vi "DataSocket Write Connections Manager.vi"(10 "URL":string, 11 "Action":enum16{"Get", "Close", "Close All"}(ring)) -> (3 "connection id":refnum<k13>)   [LabVIEW 2023, in "Reply Msg DataSocket Connections Managed.lvclass"]
uses:
  Reply Msg DataSocket Connections Managed.lvclass
  Reply Msg DataSocket Connections Managed.lvclass/Reply Msg DataSocket Connections Managed.ctl
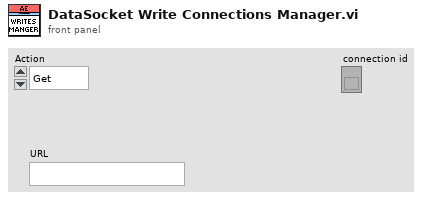
[diagram p1: front panel]
types:
  T1 = enum16{"Read", "Write", "ReadWrite", "BufferedRead", "BufferedReadWrite"}
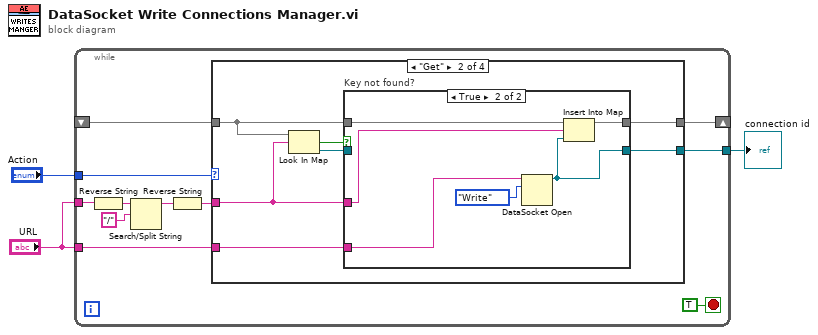
[diagram p0: block diagram]
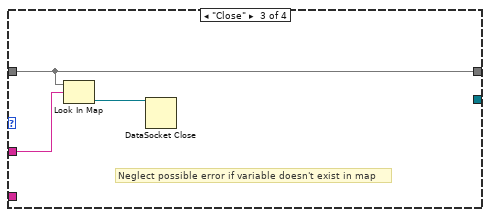
[diagram p4: hidden frame]
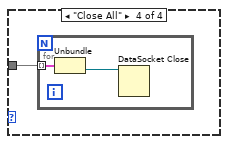
[diagram p5: hidden frame]
diagram:
  n1 = while {
    shift-right: [w12] -> _
    shift-left: _ -> [w11]
    tunnel: "URL" -> [w6]
    tunnel: [w10] -> w2
    tunnel: "Action" -> [w13]
    tunnel: "URL" -> [w4]
    stop <- TRUE stop-if-true
    n2 = Reverse String(1:w6) -> (0:w9:string)
    n3 = Search/Split String(string=w9, search string/char (-)="/") -> (substring before match=w7:string)  [unwired: 1 in, 2 out]
    n4 = Reverse String(1:w7) -> (0:w5:string)
    n5 = case shown="\"Get\"" w13 {
      tunnel: [_ w19 w30 _] -> w12
      tunnel: w11 -> [_ w20 w30 w33]
      tunnel: w5 -> [_ w18 w32 _]
      tunnel: [_ w16 _ _] -> w10
      tunnel: w4 -> [_ w15 _ _]
      frame Default {
      }
      frame "Get" {
        n6 = Look In Map(map=w20, key=w18) -> (key not found?=w21:bool, value=w17:refnum<k13>)  [unwired: 1 in]
        n7 = case "Key not found?" shown="True" w21 {
          tunnel: w20 -> [w22 w29]
          tunnel: [w22 w28] -> w19
          tunnel: w18 -> [_ w25]
          tunnel: w17 -> [w23 _]
          tunnel: [w23 w27] -> w16
          tunnel: w15 -> [_ w24]
          frame False {
          }
          frame True {
            n8 = DataSocket Open(10:T1."Write" ("mode"), 11:w24) -> (3:w27:refnum<k13>)  [unwired: 2 in, 1 out]
            n9 = Insert Into Map(map in=w29, key=w25, value=w27) -> (map out=w28:map{string, refnum<k13>})  [unwired: 2 out]
          }
        }
      }
      frame "Close" {
        # "Neglect possible error if variable doesn't exist in map"
        n10 = Look In Map(map=w30, key=w32) -> (value=w31:refnum<k13>)  [unwired: 1 in, 1 out]
        n11 = DataSocket Close(11:w31) -> ()  [unwired: 2 in, 2 out]
      }
      frame "Close All" {
        n12 = for {
          tunnel: w33 -> [w35] mode=indexing
          n13 = Unbundle(w35) -> ("connection id"=w34:refnum<k13>)  [unwired: 1 out]
          n14 = DataSocket Close(11:w34) -> ()  [unwired: 2 in, 2 out]
        }
      }
    }
  }
  "connection id" <- w2
